vi "Pad.vi"(9 "size(s)":i32, 10 "block in":u8[](array[numeric]) format="%02x", 11 "Hash Function in":refnum<class "NI_SHA-512.lvclass">) -> (2 "padded input block":u8[](array[numeric]) format="%02x", 3 "Hash Function out":refnum<class "NI_SHA-512.lvclass">)   [LabVIEW 2020, in "NI_SHA-512.lvclass"]
uses:
  <vilib>/security/Message Digest/SHA-2/SHA-512/NI_SHA-512.lvclass
  <vilib>/security/Message Digest/SHA-2/SHA-512/NI_SHA-512.lvclass/NI_SHA-512.ctl
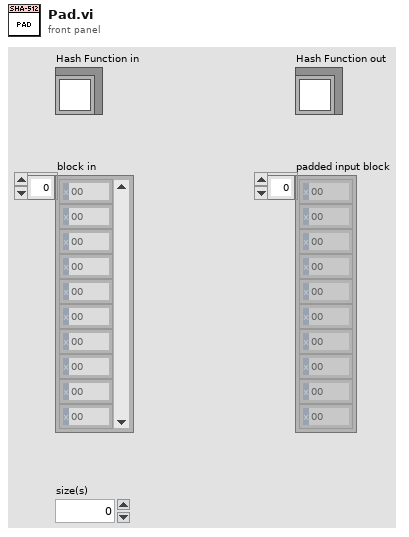
[diagram p1: front panel]
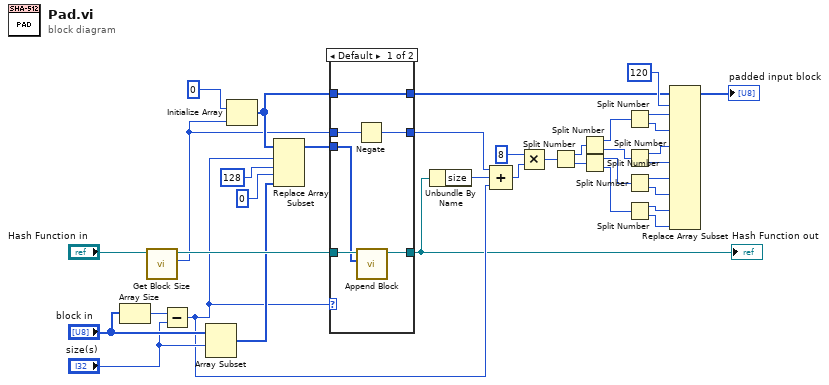
[diagram p0: block diagram]
diagram:
  n1 = Array Size(array="block in") -> (size(s)=w6:i32)
  n2 = call <vilib>:"Get Block Size.vi"("Hash Function in"="Hash Function in") -> ("block size (bytes)"=w3:i32, "Hash Function out"=w35:refnum<class "NI_SHA-512.lvclass">)  [unwired: 9 in]
  n3 = Subtract(x=w6, y="size(s)") -> (x-y=w2:i32)
  n4 = Array Subset(array="block in", index="size(s)") -> (w12:u8[])  [unwired: 1 in]
  n5 = Initialize Array(u8 0 ("index"), w3) -> (w14:u8[])
  n6 = Replace Array Subset(array=w14, new element #1=u8 128 ("index"), index #1=w2, new element #2=w12, index #2=0 ("index")) -> (w13:u8[])
  n7 = case shown="Default" w2 {
    tunnel: w13 -> [w41 w44]
    tunnel: w35 -> [w42 w43]
    tunnel: w14 -> [w39 _]
    tunnel: [w40 w43] -> w1
    tunnel: [w39 w44] -> w23
    tunnel: [w37 _] -> w4
    tunnel: w3 -> [w38 _]
    frame Default {
      n8 = Negate(x=w38) -> (-x=w37:i32)
      n9 = call <vilib>:"Append Block.vi"("block in"=w41, "Hash Function in"=w42) -> ("Hash Function out"=w40:refnum<class "NI_SHA-512.lvclass">)  [unwired: 9 in]
    }
    frame 0..111 {
    }
  }
  "Hash Function out" <- w1
  n10 = Unbundle By Name(w1) -> ("size"=w7:u64)
  n11 = Compound Arithmetic op=ADD(w4, w7, w2) -> (w5:u64)
  n12 = Multiply(x=u64 8 ("y"), y=w5) -> (x*y=w15:u64)
  n13 = Split Number(x=w15) -> (hi(x)=w16:u32, lo(x)=w17:u32)
  n14 = Split Number(x=w16) -> (hi(x)=w22:u16, lo(x)=w18:u16)
  n15 = Split Number(x=w17) -> (hi(x)=w20:u16, lo(x)=w19:u16)
  n16 = Split Number(x=w22) -> (hi(x)=w25:u8, lo(x)=w26:u8)
  n17 = Split Number(x=w18) -> (hi(x)=w27:u8, lo(x)=w28:u8)
  n18 = Split Number(x=w20) -> (hi(x)=w32:u8, lo(x)=w31:u8)
  n19 = Split Number(x=w19) -> (hi(x)=w30:u8, lo(x)=w29:u8)
  n20 = Replace Array Subset(array=w23, new element #1=w25, index #1=120 ("index"), new element #2=w26, new element #3=w27, new element #4=w28, new element #5=w32, new element #6=w31, new element #7=w30, new element #8=w29) -> (→"padded input block":u8[])  [unwired: 7 in]
